vi "VariableDelete.vi"(8 "error in (no error)":errorcluster, 10 "VariableName":string, 11 "VariablesManager in":refnum<class "VariableManager.lvclass">) -> (0 "error out":errorcluster, 3 "VariablesManager out":refnum<class "VariableManager.lvclass">)   [LabVIEW 2013, in "VariableManager.lvclass"]
doc: "Delete VariableName from database and DisplayList of all VariableGroups. \nNo operation if VariableName does not exist"
uses:
  VariableManager.lvclass
  PackedLibraries/LuaEvaluatorAPI.lvlibp/API/t_Caching_Expression_Evaluator_Methods_Table.ctl
  VariableGroup/VariableGroup.lvclass
  Variable/Variable.lvclass
  PackedLibraries/LuaEvaluatorAPI.lvlibp
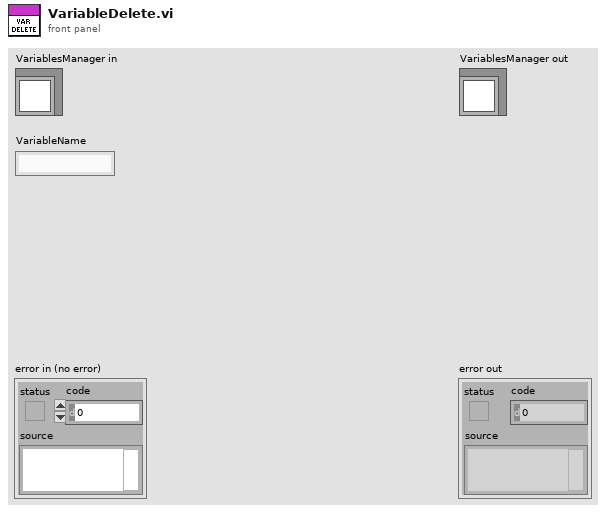
[diagram p1: front panel]
types:
  T1 = typedef "LuaEvaluatorAPI.lvlibp/t_Caching_Expression_Evaluator_Methods_Table.ctl" = enum16{"set", "get", "eval", "assign", "isvalid", "execute", "evaltable", "close"}
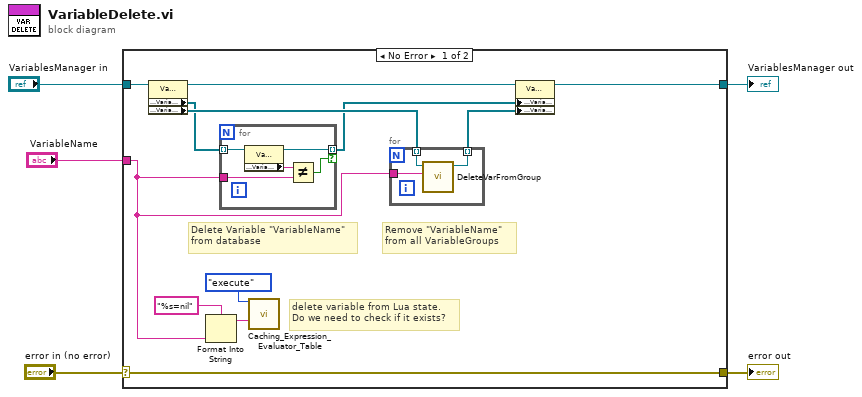
[diagram p0: block diagram]
diagram:
  n1 = case shown="No Error" "error in (no error)" {
    selector: "error in (no error)" -> [w17 w27]
    tunnel: [w17 w27] -> w4
    tunnel: [w11 w26] -> w2
    tunnel: "VariablesManager in" -> [w16 w26]
    tunnel: "VariableName" -> [w6 _]
    frame No Error {
      # "Remove \"VariableName\"\nfrom all VariableGroups"
      # "delete variable from Lua state.\nDo we need to check if it exists?"
      # "Delete Variable \"VariableName\"\nfrom database"
      n2 = property class="VariableManager.lvclass"(reference=w16) -> (reference out=w15:refnum<class "VariableManager.lvclass">, "Accessors:Variables"=w8:refnum<class "Variable.lvclass">[], "Accessors:VariableGroups"=w10:refnum<class "VariableGroup.lvclass">[])  [unwired: 1 in, 1 out]
      n3 = Format Into String(format string="%s=nil", w6) -> (resulting string=w12:string)  [unwired: 2 in, 1 out]
      n4 = for {
        tunnel: w8 -> [w22] mode=indexing
        tunnel: w6 -> [w19]
        tunnel: [w21] -> w7 mode=indexing if=w18
        n5 = property class="Variable.lvclass"(reference=w22) -> (reference out=w21:refnum<class "Variable.lvclass">, "Accessors:VariableName"=w20:string)  [unwired: 1 in, 1 out]
        n6 = Not Equal?(x=w20, y=w19) -> (x != y?=w18:bool)
      }
      n7 = call "Caching_Expression_Evaluator_Table.vi"("method"=t_Caching_Expression_Evaluator_Methods_Table."execute", "expression/scriptlet"=w12) -> ()  [unwired: 11 in, 3 out]
      n8 = for {
        tunnel: [w25] -> w9 mode=indexing
        tunnel: w6 -> [w24]
        tunnel: w10 -> [w23] mode=indexing
        n9 = call-dynamic "DeleteVarFromGroup.vi"("VariableName"=w24, "VariableGroup in"=w23) -> ("VariableGroup out"=w25:refnum<class "VariableGroup.lvclass">)  [unwired: 8 in, 1 out]
      }
      n10 = property class="VariableManager.lvclass"(reference=w15, "Accessors:Variables"=w7, "Accessors:VariableGroups"=w9) -> (reference out=w11:refnum<class "VariableManager.lvclass">)  [unwired: 1 in, 1 out]
    }
    frame Error {
    }
  }
  "error out" <- w4
  "VariablesManager out" <- w2
